vi "Heat Up Macro Main.vi"() -> ()   [LabVIEW 2016]
uses:
  Type Definitions/FilePath.ctl
  Type Definitions/Output Summary.ctl
  Type Definitions/HEWH_Type.ctl
  <vilib>/Utility/file.llb/Read From Spreadsheet File (string).vi
panel:
  out "Program Status":string
  in  "Save to Excel":bool
  in  "Exit":bool
  out "Output Summary Display":T1 {"Total Energy (W-hr)" format="%#.6g"; "HP Recovery Time (min)" format="%#.4g"; "Mid Run Evap Temp" format="%#.3g"; "Final Discharge Temp" format="%#.3g"; "EEV" format="%#_4g"; "Evap Superheat" format="%#.3g"; "Final Tank Gradient" format="%#.3g"; "UE Max Overshoot" format="%#.3g"; "Temp Drift After Recovery" format="%#.3g"; "Ambient Thermistor Accuracy" format="%#.3g"; "Water Temp Accuracy" format="%#.3g"; "Large Draw Detection" format="%#.3g"; "Gallon @ Compressor ON\nOr Time Value (Minutes)" format="%#.3g"}
  in  "Output Summary":T1 {"Total Energy (W-hr)" format="%#.6g"; "HP Recovery Time (min)" format="%#.4g"; "Mid Run Evap Temp" format="%#.3g"; "Final Discharge Temp" format="%#.3g"; "EEV" format="%#_4g"; "Evap Superheat" format="%#.3g"; "Final Tank Gradient" format="%#.3g"; "UE Max Overshoot" format="%#.3g"; "Temp Drift After Recovery" format="%#.3g"; "Ambient Thermistor Accuracy" format="%#.3g"; "Water Temp Accuracy" format="%#.3g"; "Large Draw Detection" format="%#.3g"; "Gallon @ Compressor ON\nOr Time Value (Minutes)" format="%#.3g"}
  in  "Tab Control":T3(tab)
  out "Heat Up Data":string[][](array[string])
  out "Step 1 Raw Data":string[][](array[string])
  out "Draw Flag":string[][](array[string])
  out "Large Draw":dbl[][](graph)
  out "Raw Data (Final Discharge and Compressor Shell)":string[][](array[string])
  out "Raw Data (Temp Difference)":string[][](array[string])
  out "Stabilized Condition":string[][](array[string])
  out "Tank Gradient Data":string[][](array[string])
  out "T2-Setpoint":dbl[](graph)
  out "Raw Data 2":dbl[][](array[numeric])
  out "TC Avg":cluster{"DBL":dbl[], "DBL":dbl[]}(graph)
  out "Watt Hours":cluster{"DBL":dbl[], "DBL":dbl[]}(graph)
  out "Raw Data":dbl[][](array[numeric])
  out "Evaporator Superheat":T4(graph)
  out "EEV":T4(graph)
  out "Min-Run Evap Temp (T3A)":T4(graph)
  in  "Custom Template File Path":path
  in  "Use Custom Template":bool
  in  "File Path":T5
  # "HYBRID Heat-up Macro ETP725B011"
  # "Right Click to Export to Excel"
  # "Right Click to Export to Excel"
  # "Right Click to Export to Excel"
  # "Time"
  # "Setpoint"
  # "T2"
  # "Time"
  # "Temperature"
  # "Watt Hours"
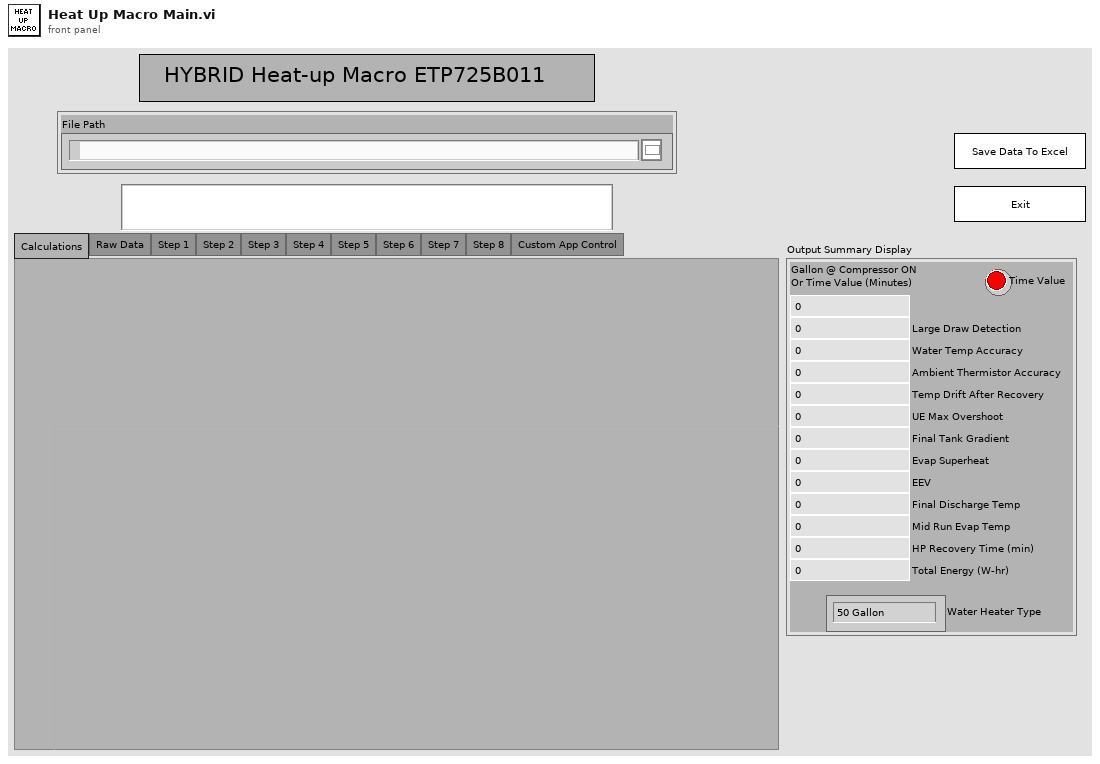
[diagram p1: front panel]
types:
  T1 = typedef "Output Summary.ctl" = cluster{"Gallon @ Compressor ON\nOr Time Value (Minutes)":dbl, "Time Value":bool, "Large Draw Detection":dbl, "Water Temp Accuracy":dbl, "Ambient Thermistor Accuracy":dbl, "Temp Drift After Recovery":dbl, "UE Max Overshoot":dbl, "Final Tank Gradient":dbl, "Evap Superheat":dbl, "EEV":u32, "Final Discharge Temp":dbl, "Mid Run Evap Temp":dbl, "HP Recovery Time (min)":dbl, "Total Energy (W-hr)":dbl, "Water Heater Type":T2}
  T2 = typedef "HEWH_Type.ctl" = enum16{"50 Gallon", "80 Gallon"}
  T3 = enum32{"Calculations", "Raw Data", "Step 1", "Step 2", "Step 3", "Step 4", "Step 5", "Step 6", "Step 7", "Step 8", "Custom App Control"}
  T4 = cluster{"X Values":dbl[], "Histogram: h(x)":i32[]}
  T5 = typedef "FilePath.ctl" = cluster{"File Path":path}
  T6 = enum32{"invalid app kind", "Development System", "Run Time System", "Student Edition", "Embedded LabVIEW", "Evaluation", "Custom"}
  T7 = enum32{"Invalid", "Standard", "Closed", "Hidden", "Minimized", "Maximized"}
  T8 = cluster{"Core":cluster{"Current VI Reference":refnum<vi>, "Close Panel on Exit?":bool}, "File Path":T5, "HeatUp Data":string[][], "Output Summary":T1}
  T9 = cluster{"Current VI Reference":refnum<vi>, "Close Panel on Exit?":bool}
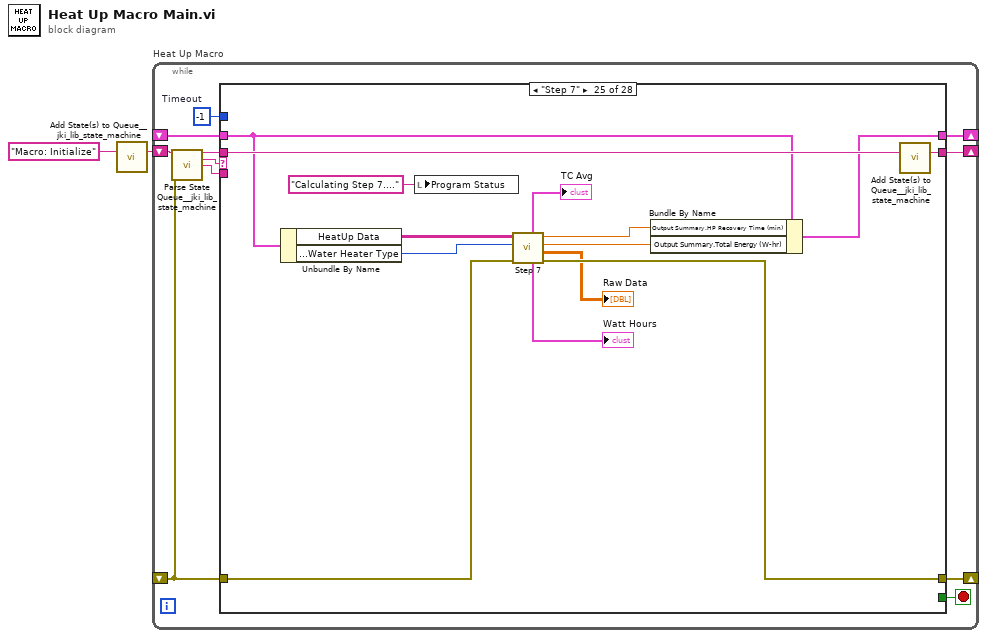
[diagram p0: block diagram]
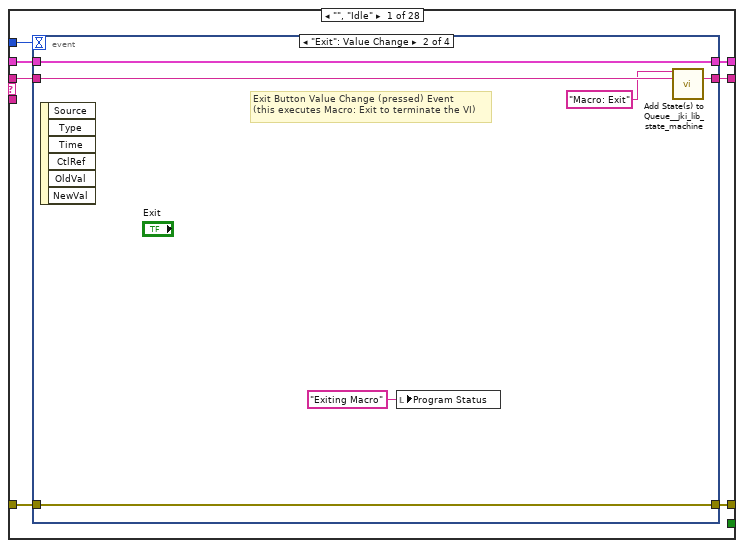
[diagram p2: hidden frame]
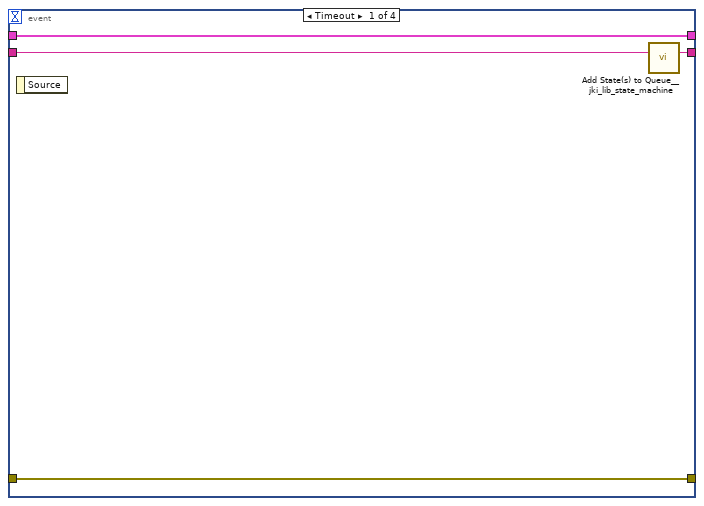
[diagram p3: hidden frame]
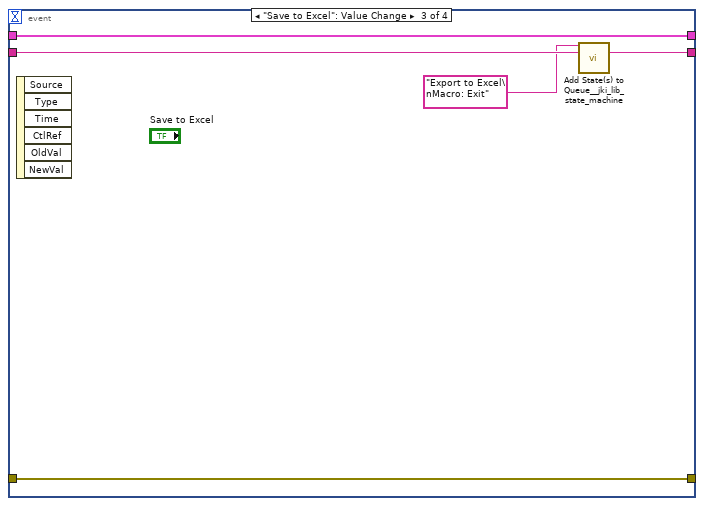
[diagram p4: hidden frame]
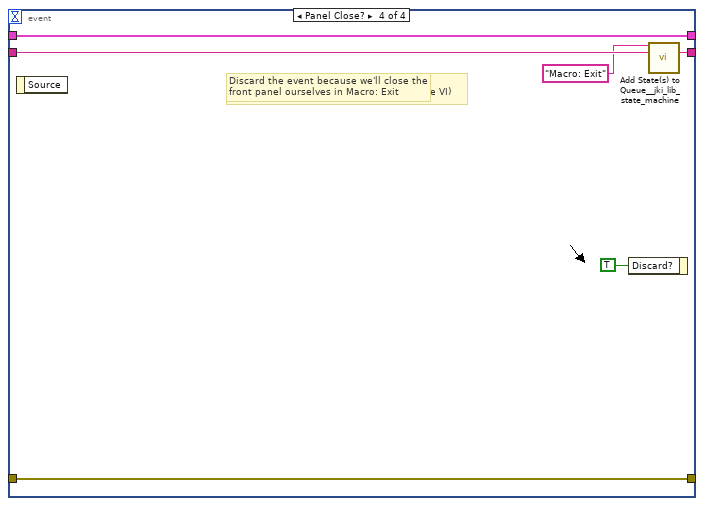
[diagram p5: hidden frame]
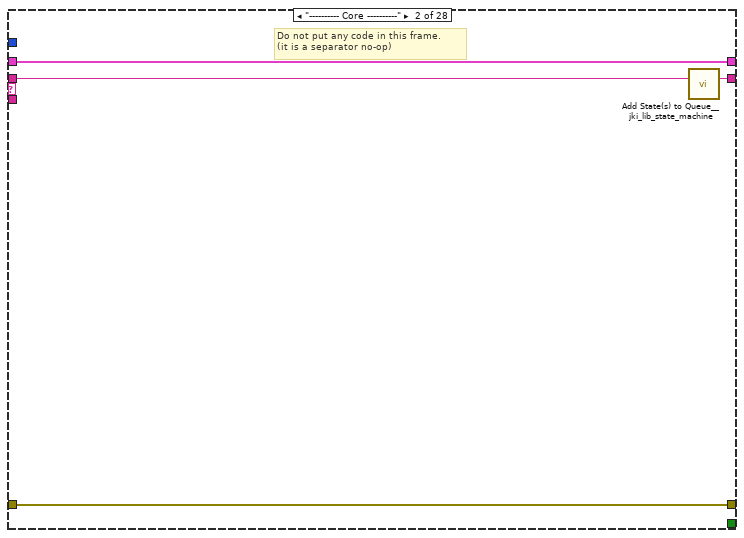
[diagram p6: hidden frame]
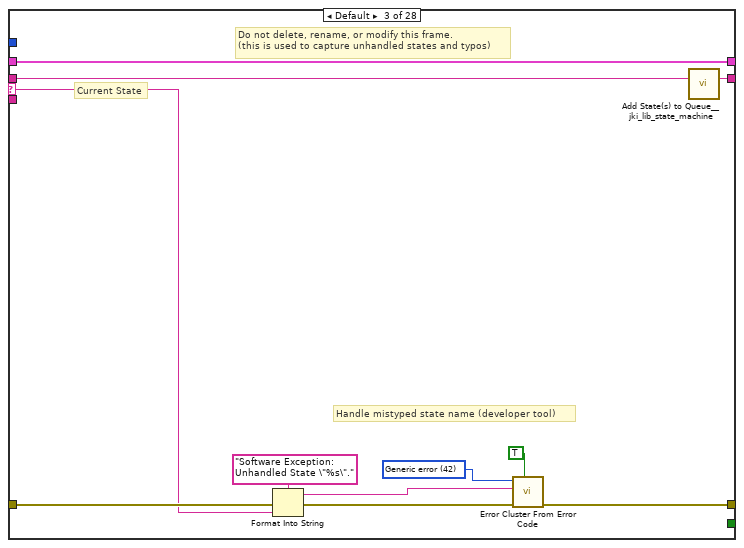
[diagram p7: hidden frame]
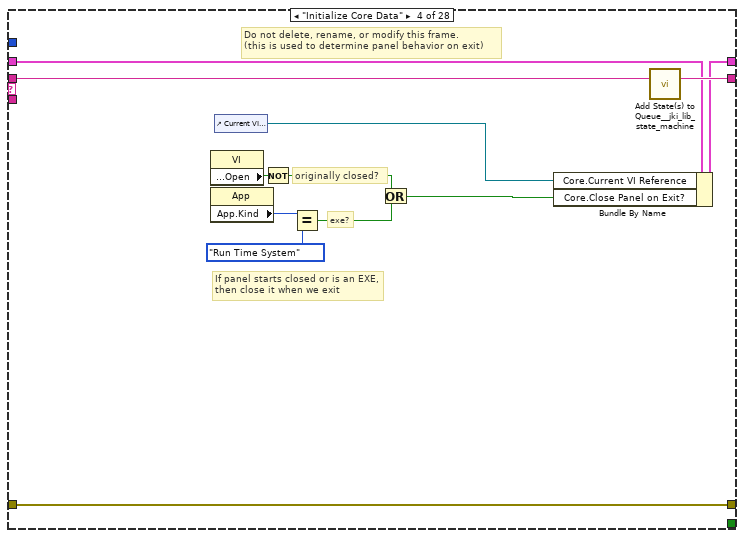
[diagram p8: hidden frame]
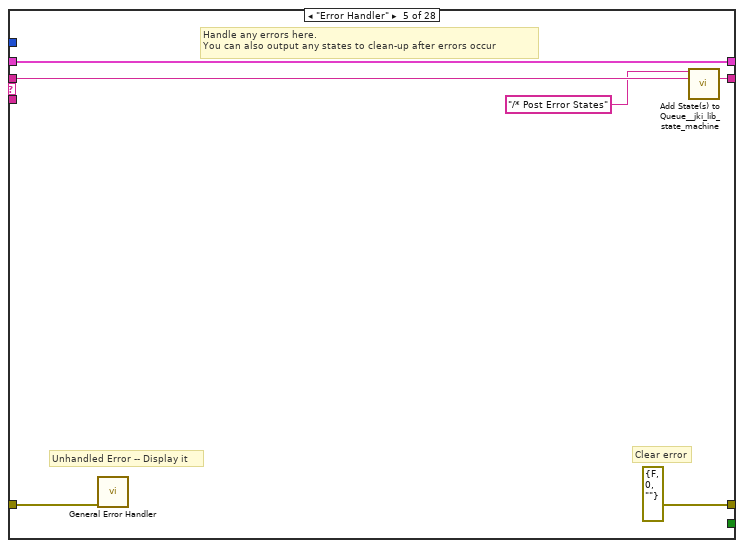
[diagram p9: hidden frame]
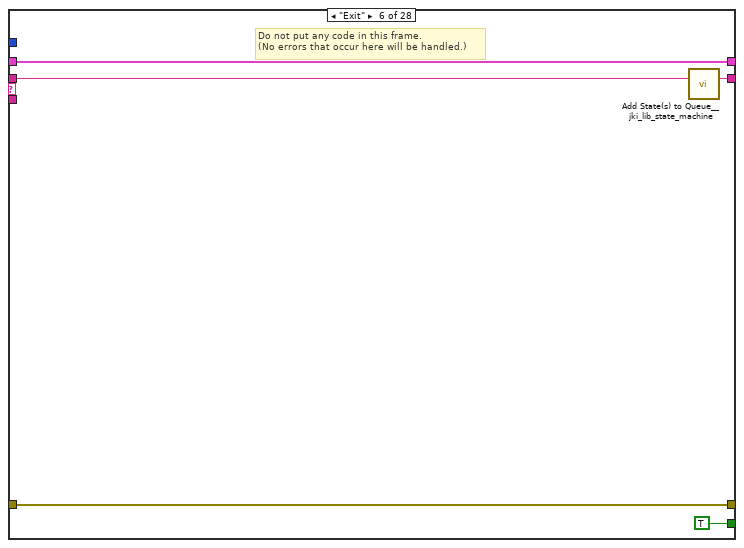
[diagram p10: hidden frame]
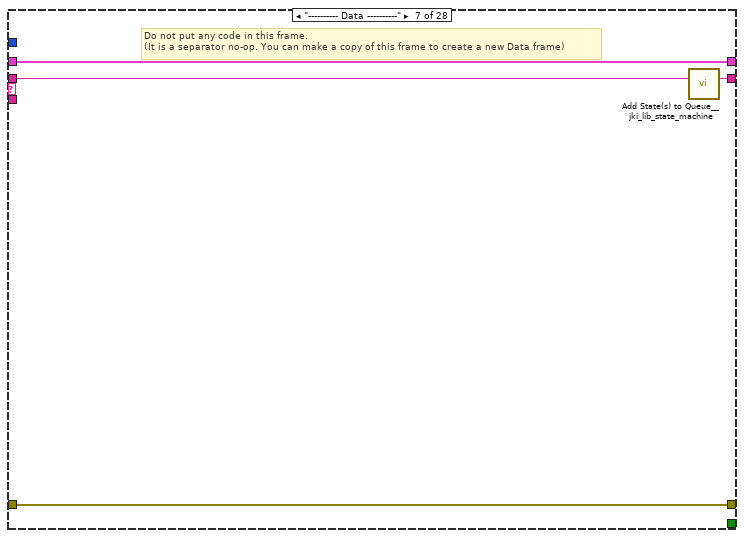
[diagram p11: hidden frame]
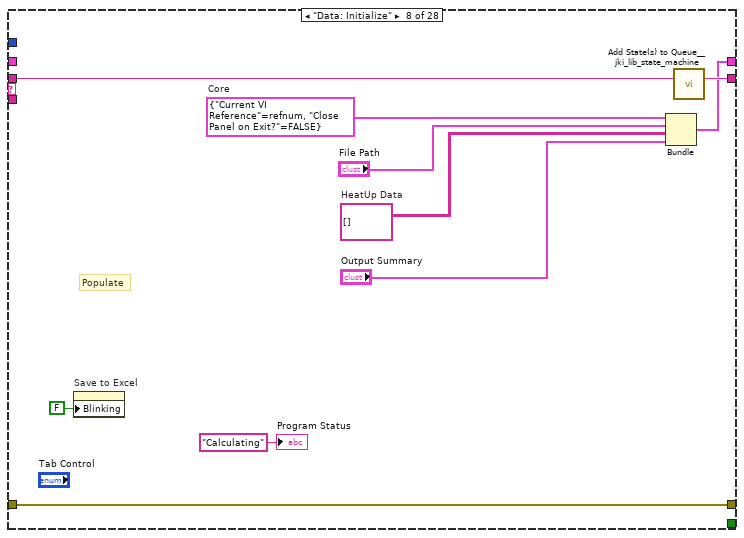
[diagram p12: hidden frame]
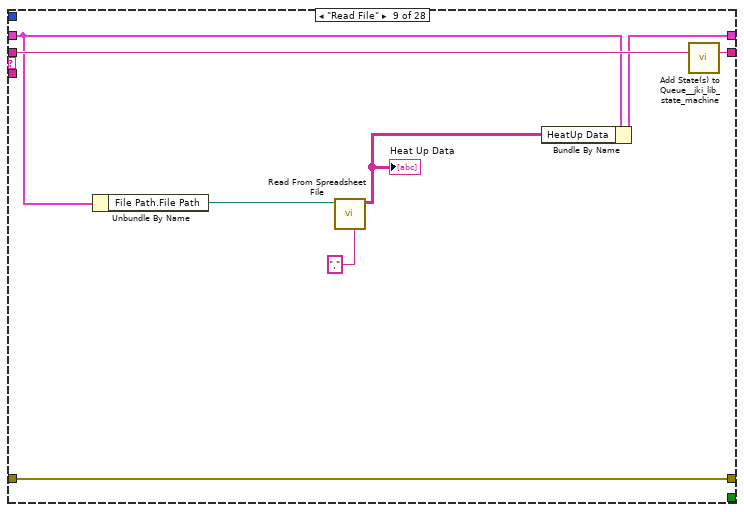
[diagram p13: hidden frame]
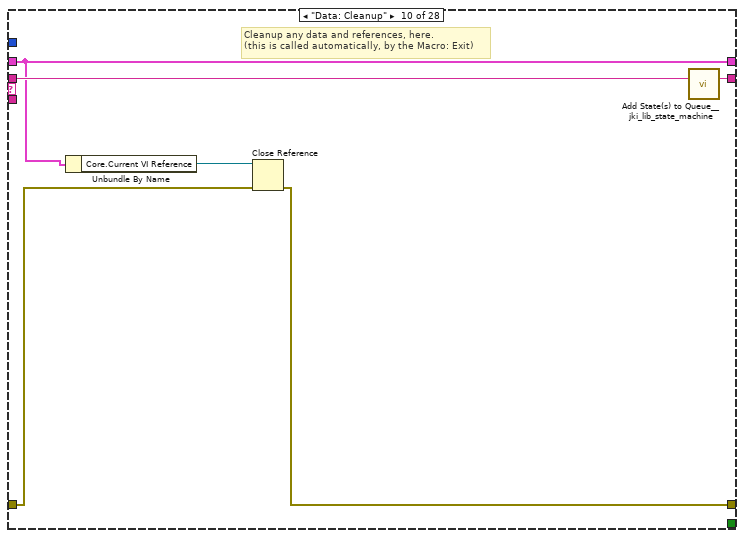
[diagram p14: hidden frame]
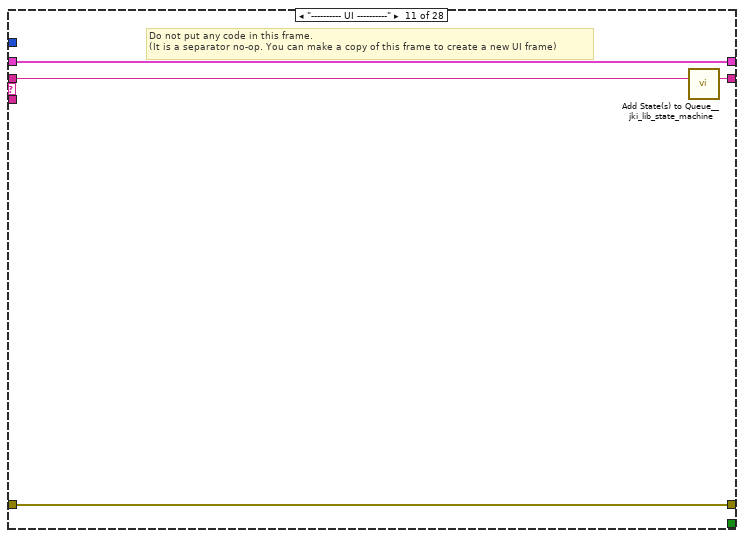
[diagram p15: hidden frame]
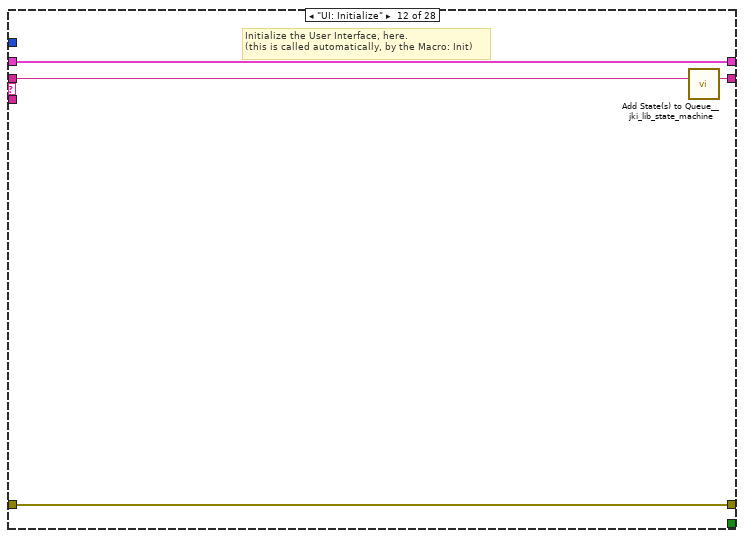
[diagram p16: hidden frame]
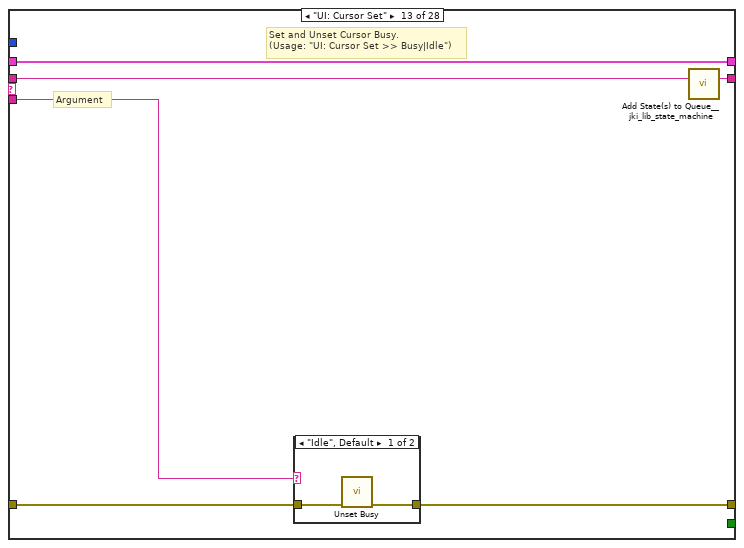
[diagram p17: hidden frame]
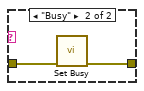
[diagram p18: hidden frame]
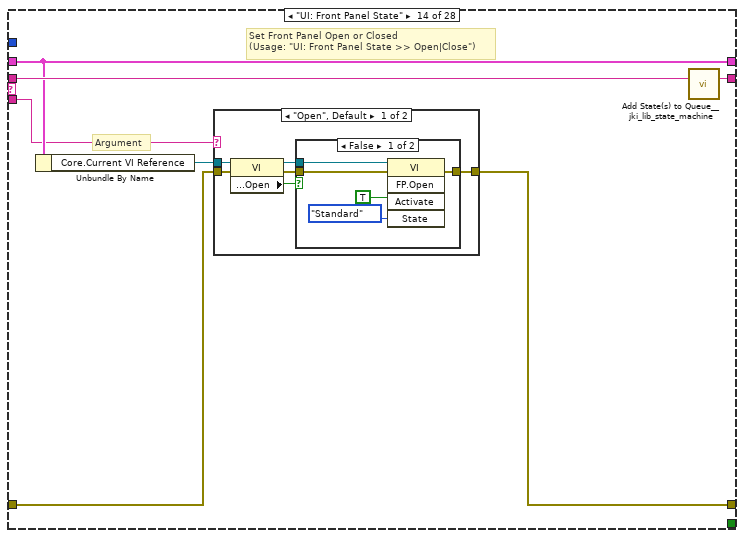
[diagram p19: hidden frame]
diagram:
  n1 = call <vilib>:"Add State(s) to Queue__jki_lib_state_machine.vi"("State(s) in (\"\")"="Macro: Initialize") -> ("States Out"=w2:string)  [unwired: 14 in]
  n2 = while "Heat Up Macro" {
    shift-right: [w6] -> _
    shift-left: _ -> [w5]
    shift-right: [w9] -> _
    shift-left: _ -> [w3]
    shift-right: [w8] -> _
    shift-left: w2 -> [w10]
    stop <- w7 stop-if-true
    w4 = -1  # Timeout
    n3 = call <vilib>:"Parse State Queue__jki_lib_state_machine.vi"("State Queue"=w10, "Error In (no error)"=w3) -> ("Remaining States"=w12:string, "Current State"=w13:string, "Arguments"=w11:string)  [unwired: 11 in]
    n4 = case shown="\"Step 7\"" w13 {
      selector: w13 -> [_ _ w46 _ _ _ _ _ _ _ _ _ _ _ _ _ _ _ _ _ _ _ _ _ _ _ _ _]
      tunnel: w12 -> [w20 w45 w50 w68 w74 w79 w83 w93 w101 w107 w111 w115 w121 w132 w158 w163 w173 w177 w189 w200 w212 w222 w233 w244 w258 w272 w278 w293]
      tunnel: w11 -> [_ _ _ _ _ _ _ _ _ _ _ _ w116 w126 _ _ _ _ _ _ _ _ _ _ _ _ _ _]
      tunnel: w5 -> [w18 w42 w48 w59 w71 w77 w80 _ w97 w105 w108 w113 w119 w128 w155 w160 w170 w174 w186 w197 w207 w218 w231 w242 w256 w270 w275 w291]
      tunnel: [w17 w43 w52 w65 errorcluster {"status"=FALSE, "code"=0, "source"=""} ("error out") w76 w81 w90 w99 w102 w109 w112 w117 w129 w156 w161 w171 w175 w181 w193 w209 w219 w226 w237 w253 w267 w276 w288] -> w9
      tunnel: w3 -> [w16 w43 w51 w65 w70 w76 w81 w90 w99 w103 w109 w112 w118 w130 w156 w161 w171 w175 w182 w194 w210 w220 w227 w238 w254 w268 w276 w289]
      tunnel: [w19 w44 w49 w67 w73 w78 w82 w92 w100 w106 w110 w114 w120 w131 w157 w162 w172 w176 w188 w199 w211 w221 w232 w243 w257 w271 w277 w292] -> w8
      tunnel: [_ _ _ _ _ TRUE _ _ _ _ _ _ _ _ _ _ _ _ _ _ _ _ _ _ _ _ _ _] -> w7
      tunnel: [w15 w42 w48 w66 w71 w77 w80 w91 w96 w105 w108 w113 w119 w128 w155 w160 w170 w174 w185 w196 w206 w217 w230 w241 w255 w269 w275 w291] -> w6
      tunnel: w4 -> [w14 _ _ _ _ _ _ _ _ _ _ _ _ _ _ _ _ _ _ _ _ _ _ _ _ _ _ _]
      frame "", "Idle" {
        n5 = event shown="[1] \"Exit\": Value Change" {
          selector: _ -> [_ _ _ _]
          dyn-events: _ -> [_ _ _ _]
          timeout: w14 -> [_ _ _ _]
          tunnel: w20 -> [w24 w30 w33 w41]
          tunnel: [w23 w29 w32 w40] -> w19
          tunnel: w18 -> [w21 w27 w35 w38]
          tunnel: [w22 w28 w34 w39] -> w17
          tunnel: w16 -> [w22 w28 w34 w39]
          tunnel: [w21 w27 w35 w38] -> w15
          event Timeout {
            n6 = event-data() -> ()  [unwired: 1 in, 1 out]
            n7 = call <vilib>:"Add State(s) to Queue__jki_lib_state_machine.vi"("State(s) in (\"\")"=w24) -> ("States Out"=w23:string)  [unwired: 14 in]
          }
          event "Exit": Value Change {
            # "Exit Button Value Change (pressed) Event\n(this executes Macro: Exit to terminate the VI)"
            n8 = event-data() -> ()  [unwired: 1 in, 6 out]
            n9 = local write "Program Status"("Exiting Macro" ("Program Status")) -> ()
            n10 = call <vilib>:"Add State(s) to Queue__jki_lib_state_machine.vi"("State(s) in Front (\"\")"="Macro: Exit", "State(s) in (\"\")"=w30) -> ("States Out"=w29:string)  [unwired: 13 in]
          }
          event "Save to Excel": Value Change {
            n11 = event-data() -> ()  [unwired: 1 in, 6 out]
            n12 = call <vilib>:"Add State(s) to Queue__jki_lib_state_machine.vi"("State(s) in Front (\"\")"="Export to Excel\nMacro: Exit", "State(s) in (\"\")"=w33) -> ("States Out"=w32:string)  [unwired: 13 in]
          }
          event Panel Close? {
            # "Discard the event because we'll close the front panel ourselves in Macro: Exit"
            # "Close Panel button (pressed) Event\n(this executes Macro: Exit to terminate the VI)"
            n13 = event-data() -> ()  [unwired: 1 in, 1 out]
            n14 = event-data("Discard?"=TRUE) -> ()  [unwired: 1 in, 1 out]
            n15 = call <vilib>:"Add State(s) to Queue__jki_lib_state_machine.vi"("State(s) in Front (\"\")"="Macro: Exit", "State(s) in (\"\")"=w41) -> ("States Out"=w40:string)  [unwired: 13 in]
          }
        }
      }
      frame "---------- Core ----------" {
        # "Do not put any code in this frame.\n(it is a separator no-op)"
        n16 = call <vilib>:"Add State(s) to Queue__jki_lib_state_machine.vi"("State(s) in (\"\")"=w45) -> ("States Out"=w44:string)  [unwired: 14 in]
      }
      frame Default {
        w55 = 42 items=["No error", "Argument error", "Memory is full", "Out of zone", "End of file", "File already open", "Generic file I/O error", "File not found", "File permission error", "Disk is full", "Duplicate path", "Too many files open", "System feature not enabled", "Resource file not found", "Cannot add resource", "Resource not found", "Image not found", "Image memory error", "Pen does not exist", "Config type invalid", "Config token not found", "Config parse error", "Config memory error", "Bad external code format", "Bad external code offset", "External code not present", "Null window", "Destroy window error", "Null menu", "Print aborted", "Bad print record", "Print driver error", "Windows error during printing", "Memory error during printing", "Print dialog error", "Generic print error", "Invalid device refnum", "Device not found", "Device parameter error", "Device unit error", "Cannot open device", "Device call aborted", "Generic error", "Cancelled by user", "Object ID too low", "Object ID too high", "Object not in heap", "Unknown heap", "Unknown object (invalid DefProc)", "Unknown object (DefProc not in table)", "Message out of range", "Invalid (null) method", "Unknown message", "Manager call not supported", "Bad address", "Network operation in progress", "Network operation timed out", "Connection is busy", "Network attribute not supported", "Network error", "Address in use", "System out of memory", "Connection aborted", "Connection refused", "Not connected", "Already connected", "Connection closed", "Initialization error (interapplication manager)", "Bad occurrence", "Wait on unbound occurrence handler", "Occurrence queue overflow", "Datalog type conflict", "Unused", "Unrecognized type (interapplication manager)", "Memory corrupt", "Failed to make temporary DLL", "Old CIN version", "Drag socket not found", "Failed to load drop-object", "Failed to register OLE object", "Failed to release OLE object", "Format specifier type mismatch", "Unknown format specifier", "Too few format specifiers", "Too many format specifiers", "Scan failed", "Newer CIN version", "Error converting to variant", "Runtime menu error", "Password tampered", "Variant attribute not found", "Incompatible variant data type", "Event data is not available", "Event Store is not present", "Occurrence is not found", "Event Queue is not created", "Event info is not available", "Refnum passed is NULL", "Error retrieving Class GUID", "Error retrieving CoClass GUID", "Error retrieving TypeLib GUID.", "Bad built application magic bytes.", "Specific driver is different from the specific driver associated with the Logical Name.", "There is no session opened to the class driver.", "Max Error", "MAX - Error with config objects", "MAX - Error loading configuration", "MAX - Group not supported"]
        # "Current State"
        # "Do not delete, rename, or modify this frame.\n(this is used to capture unhandled states and typos)"
        # "Handle mistyped state name (developer tool)"
        n17 = Format Into String(format string="Software Exception: Unhandled State \"%s\"." ("message"), error in=w51, w46) -> (resulting string=w54:string, error out=w53:errorcluster)  [unwired: 1 in]
        n18 = call <vilib>:"Error Cluster From Error Code.vi"("show call chain? (False)"=TRUE, "error in (no error)"=w53, "error message (\"\")"=w54, "error code (0)"=w55) -> ("error out"=w52:errorcluster)  [unwired: 5 in]
        n19 = call <vilib>:"Add State(s) to Queue__jki_lib_state_machine.vi"("State(s) in (\"\")"=w50) -> ("States Out"=w49:string)  [unwired: 14 in]
      }
      frame "Initialize Core Data" {
        # "Do not delete, rename, or modify this frame.\n(this is used to determine panel behavior on exit)"
        # "originally closed?"
        # "exe?"
        # "If panel starts closed or is an EXE, then close it when we exit"
        n20 = property class="VI"() -> ("Front Panel.Open"=w64:bool)  [unwired: 2 in, 2 out]
        n21 = property class="App"() -> ("App.Kind"=w63:T6)  [unwired: 2 in, 2 out]
        n22 = control-ref of="Current VI Reference"() -> (w57:refnum<vi>)
        n23 = Not(x=w64) -> (.not. x?=w61:bool)
        n24 = Equal?(x=w63, y=T6."Run Time System" ("Application:Kind")) -> (x = y?=w60:bool)
        n25 = Or(x=w61, y=w60) -> (x .or. y?=w58:bool)
        n26 = Bundle By Name(cluster=w59, "Core.Current VI Reference"=w57, "Core.Close Panel on Exit?"=w58) -> (w66:T8)
        n27 = call <vilib>:"Add State(s) to Queue__jki_lib_state_machine.vi"("State(s) in (\"\")"=w68) -> ("States Out"=w67:string)  [unwired: 14 in]
      }
      frame "Error Handler" {
        # "Unhandled Error -- Display it"
        # "Handle any errors here.\nYou can also output any states to clean-up after errors occur"
        # "Clear error"
        n28 = call <vilib>:"General Error Handler.vi"("error in (no error)"=w70) -> ()  [unwired: 10 in, 5 out]
        n29 = call <vilib>:"Add State(s) to Queue__jki_lib_state_machine.vi"("State(s) in Front (\"\")"="/* Post Error States", "State(s) in (\"\")"=w74) -> ("States Out"=w73:string)  [unwired: 13 in]
      }
      frame "Exit" {
        # "Do not put any code in this frame.\n(No errors that occur here will be handled.)"
        n30 = call <vilib>:"Add State(s) to Queue__jki_lib_state_machine.vi"("State(s) in (\"\")"=w79) -> ("States Out"=w78:string)  [unwired: 14 in]
      }
      frame "---------- Data ----------" {
        # "Do not put any code in this frame.\n(It is a separator no-op. You can make a copy of this frame to create a new Data frame)"
        n31 = call <vilib>:"Add State(s) to Queue__jki_lib_state_machine.vi"("State(s) in (\"\")"=w83) -> ("States Out"=w82:string)  [unwired: 14 in]
      }
      frame "Data: Initialize" {
        w87 = string[][] []  # HeatUp Data
        w89 = T9 {"Current VI Reference"=refnum, "Close Panel on Exit?"=FALSE}  # Core
        # "Populate"
        n32 = property on="Save to Excel" class="Bool"("Blinking"=FALSE) -> ()  [unwired: 2 in, 2 out]
        n33 = Bundle("Core"=w89, "File Path"="File Path", "HeatUp Data"=w87, "Output Summary"="Output Summary") -> (w91:T8)  [unwired: 1 in]
        n34 = call <vilib>:"Add State(s) to Queue__jki_lib_state_machine.vi"("State(s) in (\"\")"=w93) -> ("States Out"=w92:string)  [unwired: 14 in]
        "Program Status" <- "Calculating" ("Program Status")
      }
      frame "Read File" {
        n35 = Unbundle By Name(w97) -> ("File Path.File Path"=w98:path)
        n36 = call-poly <vilib>:"Read From Spreadsheet File.vi"("delimiter (\\t)"="," ("delimiter (\\t)"), "file path (dialog if empty)"=w98) -> ("all rows"=w95:string[][])  [unwired: 5 in, 4 out]
        "Heat Up Data" <- w95
        n37 = Bundle By Name(cluster=w97, "HeatUp Data"=w95) -> (w96:T8)
        n38 = call <vilib>:"Add State(s) to Queue__jki_lib_state_machine.vi"("State(s) in (\"\")"=w101) -> ("States Out"=w100:string)  [unwired: 14 in]
      }
      frame "Data: Cleanup" {
        # "Cleanup any data and references, here.\n(this is called automatically, by the Macro: Exit)"
        n39 = Unbundle By Name(w105) -> ("Core.Current VI Reference"=w104:refnum<vi>)
        n40 = Close Reference(reference=w104, error in (no error)=w103) -> (error out=w102:errorcluster)
        n41 = call <vilib>:"Add State(s) to Queue__jki_lib_state_machine.vi"("State(s) in (\"\")"=w107) -> ("States Out"=w106:string)  [unwired: 14 in]
      }
      frame "---------- UI ----------" {
        # "Do not put any code in this frame.\n(It is a separator no-op. You can make a copy of this frame to create a new UI frame)"
        n42 = call <vilib>:"Add State(s) to Queue__jki_lib_state_machine.vi"("State(s) in (\"\")"=w111) -> ("States Out"=w110:string)  [unwired: 14 in]
      }
      frame "UI: Initialize" {
        # "Initialize the User Interface, here.\n(this is called automatically, by the Macro: Init)"
        n43 = call <vilib>:"Add State(s) to Queue__jki_lib_state_machine.vi"("State(s) in (\"\")"=w115) -> ("States Out"=w114:string)  [unwired: 14 in]
      }
      frame "UI: Cursor Set" {
        # "Argument"
        # "Set and Unset Cursor Busy.\n(Usage: \"UI: Cursor Set >> Busy|Idle\")"
        n44 = case shown="\"Idle\", Default" w116 {
          tunnel: w118 -> [w123 w125]
          tunnel: [w122 w124] -> w117
          frame "Idle", Default {
            n45 = call <vilib>:"Unset Busy.vi"("error in (no error)"=w123) -> ("error out"=w122:errorcluster)  [unwired: 10 in]
          }
          frame "Busy" {
            n46 = call <vilib>:"Set Busy.vi"("error in (no error)"=w125) -> ("error out"=w124:errorcluster)  [unwired: 9 in, 1 out]
          }
        }
        n47 = call <vilib>:"Add State(s) to Queue__jki_lib_state_machine.vi"("State(s) in (\"\")"=w121) -> ("States Out"=w120:string)  [unwired: 14 in]
      }
      frame "UI: Front Panel State" {
        # "Argument"
        # "Set Front Panel Open or Closed\n(Usage: \"UI: Front Panel State >> Open|Close\")"
        n48 = Unbundle By Name(w128) -> ("Core.Current VI Reference"=w127:refnum<vi>)
        n49 = case shown="\"Open\", Default" w126 {
          tunnel: w130 -> [w136 w149]
          tunnel: [w138 w150] -> w129
          tunnel: w127 -> [w137 w147]
          frame "Open", Default {
            n50 = property class="VI"(reference=w137, error in=w136) -> (reference out=w134:refnum<vi>, error out=w135:errorcluster, "Front Panel.Open"=w133:bool)
            n51 = case shown="False" w133 {
              tunnel: [w141 w144] -> w138
              tunnel: w135 -> [w140 w144]
              tunnel: w134 -> [w139 _]
              frame False {
                n52 = invoke class="VI" method="FP.Open"(reference=w139, error in=w140, "Activate"=TRUE, "State"=T7."Standard") -> (error out=w141:errorcluster)  [unwired: 1 in, 4 out]
              }
              frame True {
              }
            }
          }
          frame "Close" {
            n53 = property class="VI"(reference=w147, error in=w149) -> (reference out=w146:refnum<vi>, error out=w148:errorcluster, "Front Panel.Open"=w145:bool)
            n54 = case shown="True" w145 {
              tunnel: [w151 w154] -> w150
              tunnel: w148 -> [w151 w153]
              tunnel: w146 -> [_ w152]
              frame False {
              }
              frame True {
                n55 = invoke class="VI" method="FP.Close"(reference=w152, error in=w153) -> (error out=w154:errorcluster)  [unwired: 1 in, 2 out]
              }
            }
          }
        }
        n56 = call <vilib>:"Add State(s) to Queue__jki_lib_state_machine.vi"("State(s) in (\"\")"=w132) -> ("States Out"=w131:string)  [unwired: 14 in]
      }
      frame "---------- Macro ----------" {
        # "Do not put any code in this frame.\n(It is a separator no-op. You can make a copy of this frame to create a new Macro frame)"
        n57 = call <vilib>:"Add State(s) to Queue__jki_lib_state_machine.vi"("State(s) in (\"\")"=w158) -> ("States Out"=w157:string)  [unwired: 14 in]
      }
      frame "Macro: Initialize" {
        w159 = "Data: Initialize\nInitialize Core Data\nUI: Initialize\nUI: Front Panel State >> Open\nRead File\nStep 1\nStep 2\nStep 3\nStep 4\nStep 5\nStep 6\nStep 7\nStep 8\nDisplay"  # Data: Initialize Initialize Core Data UI: Initialize UI: Front Panel State >> Open Read File Step 1 Step 2 Step 3 Step 4 Step 5 Step 6 Step 7 Step 8 Display
        # "Initialization Macro\n(This is called once, when the VI starts)"
        n58 = call <vilib>:"Add State(s) to Queue__jki_lib_state_machine.vi"("State(s) in Front (\"\")"=w159, "State(s) in (\"\")"=w163) -> ("States Out"=w162:string)  [unwired: 13 in]
      }
      frame "Macro: Exit" {
        # "Exit Macro\n(This is called once, when the VI exits)"
        n59 = Unbundle By Name(w170) -> ("Core.Close Panel on Exit?"=w169:bool)
        n60 = Select(t="UI: Front Panel State >> Open", s=w169, f="") -> (s? t:f=w166:string)
        n61 = call <vilib>:"Add State(s) to Queue__jki_lib_state_machine.vi"("State(s) in (\"\")"=w166, "State(s) at Back (\"\")"="Data: Cleanup\nExit") -> ("States Out"=w164:string)  [unwired: 13 in]
        n62 = call <vilib>:"Add State(s) to Queue__jki_lib_state_machine.vi"("State(s) in Front (\"\")"=w164, "State(s) in (\"\")"=w173) -> ("States Out"=w172:string)  [unwired: 13 in]
      }
      frame "---------- New Category ----------" {
        # "Template Separator\n(You can make a copy of, or modify, this frame)"
        n63 = call <vilib>:"Add State(s) to Queue__jki_lib_state_machine.vi"("State(s) in (\"\")"=w177) -> ("States Out"=w176:string)  [unwired: 14 in]
      }
      frame "Step 1" {
        # "After 10-gallon draw- Determine Time or\n Gallons before lower heat source energizes\n (min)"
        n64 = Unbundle By Name(w186) -> ("HeatUp Data"=w187:string[][])
        n65 = call "Step 1.vi"("error in (no error)"=w182, "HeatUp Data in"=w187) -> ("error out"=w181:errorcluster, "Water Heater Type"=w180:T2, "Time"=w183:bool, "Gallon @ Compressor ON\nOr Time Value (Minutes)"=w184:dbl, "HeatUp Data in 2"=→"Step 1 Raw Data":string[][])  [unwired: 5 in]
        n66 = Bundle By Name(cluster=w186, "Output Summary.Gallon @ Compressor ON\nOr Time Value (Minutes)"=w184, "Output Summary.Time Value"=w183, "Output Summary.Water Heater Type"=w180) -> (w185:T8)
        n67 = local write "Program Status"("Calculating Step 1...." ("Program Status")) -> ()
        n68 = call <vilib>:"Add State(s) to Queue__jki_lib_state_machine.vi"("State(s) in (\"\")"=w189) -> ("States Out"=w188:string)  [unwired: 14 in]
      }
      frame "Step 2" {
        # "Large Draw Detection"
        n69 = Unbundle By Name(w197) -> ("HeatUp Data"=w198:string[][])
        n70 = call "Step 2.vi"("error in (no error)"=w194, "HeatUp Data in"=w198) -> ("error out"=w193:errorcluster, "Large Draw"=→"Large Draw":dbl[][], "Draw Flag"=→"Draw Flag":string[][], "Large Draw Flag Gallons"=w195:dbl)  [unwired: 6 in]
        n71 = Bundle By Name(cluster=w197, "Output Summary.Large Draw Detection"=w195) -> (w196:T8)
        n72 = local write "Program Status"("Calculating Step 2...." ("Program Status")) -> ()
        n73 = call <vilib>:"Add State(s) to Queue__jki_lib_state_machine.vi"("State(s) in (\"\")"=w200) -> ("States Out"=w199:string)  [unwired: 14 in]
      }
      frame "Step 3" {
        # "Water Temp Accuracy to Setpoint"
        n74 = Unbundle By Name(w207) -> ("HeatUp Data"=w208:string[][])
        n75 = call "Step 3.vi"("error in (no error)"=w210, "HeatUp Data in"=w208) -> ("error out"=w209:errorcluster, "Final Discharge Temperature"=w204:dbl, "Max Temp Difference"=w205:dbl, "Raw Data (Final Discharge and Compressor Shell)"=→"Raw Data (Final Discharge and Compressor Shell)":string[][], "Raw Data (Temp Difference)"=→"Raw Data (Temp Difference)":string[][])  [unwired: 5 in]
        n76 = Bundle By Name(cluster=w207, "Output Summary.Water Temp Accuracy"=w205, "Output Summary.Final Discharge Temp"=w204) -> (w206:T8)
        n77 = local write "Program Status"("Calculating Step 3...." ("Program Status")) -> ()
        n78 = call <vilib>:"Add State(s) to Queue__jki_lib_state_machine.vi"("State(s) in (\"\")"=w212) -> ("States Out"=w211:string)  [unwired: 14 in]
      }
      frame "Step 4" {
        n79 = Unbundle By Name(w218) -> ("HeatUp Data"=w215:string[][])
        n80 = call "Step 4.vi"("error in (no error)"=w220, "HeatUp Data in"=w215) -> ("error out"=w219:errorcluster, "Stabilized Condition"=→"Stabilized Condition":string[][], "Max Temp Difference"=w216:dbl)  [unwired: 7 in]
        n81 = Bundle By Name(cluster=w218, "Output Summary.Ambient Thermistor Accuracy"=w216) -> (w217:T8)
        n82 = local write "Program Status"("Calculating Step 4...." ("Program Status")) -> ()
        n83 = call <vilib>:"Add State(s) to Queue__jki_lib_state_machine.vi"("State(s) in (\"\")"=w222) -> ("States Out"=w221:string)  [unwired: 14 in]
      }
      frame "Step 5" {
        # "Temperature Drift after recorvery (F)\n1. Looks at end points"
        n84 = Unbundle By Name(w231) -> ("HeatUp Data"=w229:string[][])
        n85 = call "Step 5.vi"("error in (no error)"=w227, "HeatUp Data in"=w229) -> ("error out"=w226:errorcluster, "Tank Gradient"=w225:dbl, "Max Temp Drift"=w228:dbl, "Tank Gradient Data"=→"Tank Gradient Data":string[][])  [unwired: 6 in]
        n86 = Bundle By Name(cluster=w231, "Output Summary.Temp Drift After Recovery"=w228, "Output Summary.Final Tank Gradient"=w225) -> (w230:T8)
        n87 = local write "Program Status"("Calculating Step 5...." ("Program Status")) -> ()
        n88 = call <vilib>:"Add State(s) to Queue__jki_lib_state_machine.vi"("State(s) in (\"\")"=w233) -> ("States Out"=w232:string)  [unwired: 14 in]
      }
      frame "Step 6" {
        n89 = Unbundle By Name(w242) -> ("HeatUp Data"=w240:string[][])
        n90 = call "Step 6.vi"("error in (no error)"=w238, "HeatUp Data in"=w240) -> ("error out"=w237:errorcluster, "T2-Setpoint"=→"T2-Setpoint":dbl[], "Raw Data"=→"Raw Data 2":dbl[][], "Overshoot"=w239:dbl)  [unwired: 6 in]
        n91 = Bundle By Name(cluster=w242, "Output Summary.UE Max Overshoot"=w239) -> (w241:T8)
        n92 = local write "Program Status"("Calculating Step 6...." ("Program Status")) -> ()
        n93 = call <vilib>:"Add State(s) to Queue__jki_lib_state_machine.vi"("State(s) in (\"\")"=w244) -> ("States Out"=w243:string)  [unwired: 14 in]
      }
      frame "Step 7" {
        n94 = Unbundle By Name(w256) -> ("HeatUp Data"=w252:string[][], "Output Summary.Water Heater Type"=w249:T2)
        n95 = local write "Program Status"("Calculating Step 7...." ("Program Status")) -> ()
        n96 = call "Step 7.vi"("error in (no error)"=w254, "Water Heater Type"=w249, "HeatUp Data in"=w252) -> ("error out"=w253:errorcluster, "110-130 Array"=→"Raw Data":dbl[][], "Total Energy Expended (W-hr)"=w250:dbl, "HP Recovery Time"=w251:dbl, "Watt Hours"=→"Watt Hours":cluster{"DBL":dbl[], "DBL":dbl[]}, "TC Avg"=→"TC Avg":cluster{"DBL":dbl[], "DBL":dbl[]})  [unwired: 3 in]
        n97 = Bundle By Name(cluster=w256, "Output Summary.HP Recovery Time (min)"=w251, "Output Summary.Total Energy (W-hr)"=w250) -> (w255:T8)
        n98 = call <vilib>:"Add State(s) to Queue__jki_lib_state_machine.vi"("State(s) in (\"\")"=w258) -> ("States Out"=w257:string)  [unwired: 14 in]
      }
      frame "Step 8" {
        n99 = Unbundle By Name(w270) -> ("HeatUp Data"=w266:string[][])
        n100 = call "Step 8.vi"("error in (no error)"=w268, "HeatUp Data in"=w266) -> ("error out"=w267:errorcluster, 1:"Min-Run Evap Temp (T3A)"=w263:dbl, 2:"EEV"=w264:u32, "Evaporator Superheat (Deg F)"=w265:dbl, "Evaporator Superheat"=→"Evaporator Superheat":T4, 5:"Min-Run Evap Temp (T3A)"=→"Min-Run Evap Temp (T3A)":T4, 7:"EEV"=→"EEV":T4)  [unwired: 3 in]
        n101 = Bundle By Name(cluster=w270, "Output Summary.Evap Superheat"=w265, "Output Summary.EEV"=w264, "Output Summary.Mid Run Evap Temp"=w263) -> (w269:T8)
        n102 = local write "Program Status"("Calculating Step 8...." ("Program Status")) -> ()
        n103 = call <vilib>:"Add State(s) to Queue__jki_lib_state_machine.vi"("State(s) in (\"\")"=w272) -> ("States Out"=w271:string)  [unwired: 14 in]
      }
      frame "Display" {
        n104 = Unbundle By Name(w275) -> ("Output Summary"=→"Output Summary Display":T1)
        n105 = local write "Program Status"("Press Save to Excel or Exit" ("Program Status")) -> ()
        n106 = call <vilib>:"Add State(s) to Queue__jki_lib_state_machine.vi"("State(s) in (\"\")"=w278) -> ("States Out"=w277:string)  [unwired: 14 in]
      }
      frame "Export to Excel" {
        n107 = Unbundle By Name(w291) -> ("Output Summary"=w286:T1, "File Path.File Path"=w290:path, "HeatUp Data"=w287:string[][])
        n108 = Two Button Dialog(message="How would you like the data saved?\nOption 1: Create a new save location\nCancel. I made a mistake! Ahh :)", 1:"Cancel" ("F button name (\"Cancel\")"), 2:"Option 1:" ("T button name (\"OK\")")) -> (T button?=w279:bool)
        n109 = case shown="False" "Use Custom Template" {
          tunnel: [w302 w303] -> w285
          tunnel: "Custom Template File Path" -> [_ w303]
          frame False {
            n110 = call "Template Path.vi"() -> ("path"=w302:path)  [unwired: 11 in]
          }
          frame True {
          }
        }
        n111 = case shown="True" w279 {
          tunnel: w290 -> [_ _]
          tunnel: w289 -> [w297 w301]
          tunnel: [w296 w301] -> w288
          tunnel: w287 -> [w298 _]
          tunnel: w286 -> [w299 _]
          tunnel: w285 -> [w295 _]
          frame True {
            n112 = local write "Program Status"("Saving To Excel" ("Program Status")) -> ()
            n113 = call "Save To Excel.vi"("Excel Template"=w295, "Output Summary Display"=w299, "error in (no error)"=w297, "HeatUp Data"=w298) -> ("error out"=w296:errorcluster)  [unwired: 7 in]
          }
          frame False {
            n114 = local write "Program Status"("Cancelling Save" ("Program Status")) -> ()
          }
        }
        n115 = disable-structure shown="Disabled" {
          frame Disabled {
            n116 = call "Save To Excel.vi"() -> ()  [unwired: 11 in, 1 out]
          }
          frame Enabled {
          }
        }
        n117 = call <vilib>:"Add State(s) to Queue__jki_lib_state_machine.vi"("State(s) in (\"\")"=w293) -> ("States Out"=w292:string)  [unwired: 14 in]
      }
    }
  }
